vi "CreateRecordingFolder.vi"(0 "Data folder":path, 1 "mouseNumber":i32, 2 "sessionID":string, 4 "Google Drive":bool) -> (5 "Recording Path":path)   [LabVIEW 2013]
panel:
  # "INPUTS"
  # "OUTPUTS"
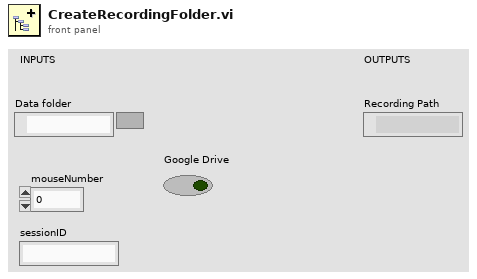
[diagram p1: front panel]
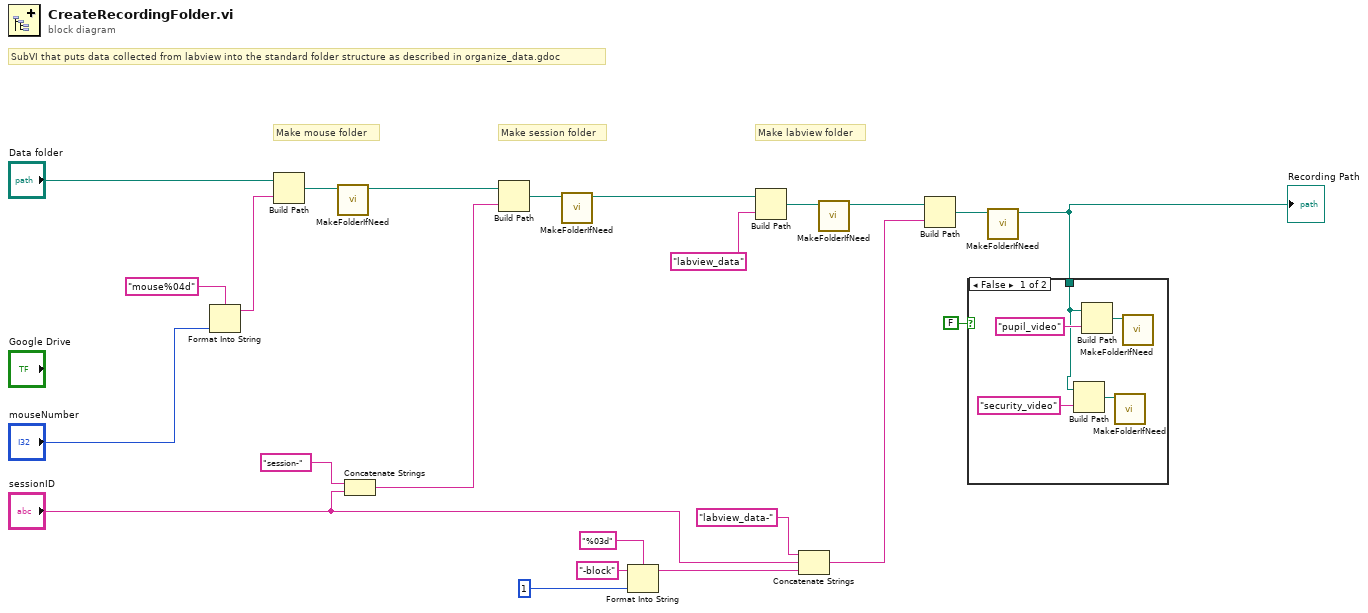
[diagram p0: block diagram]
diagram:
  # "SubVI that puts data collected from labview into the standard folder structure as described in organize_data.gdoc"
  # "Make labview folder"
  # "Make session folder"
  # "Make mouse folder"
  n1 = Format Into String(format string="mouse%04d", "mouseNumber") -> (resulting string=w16:string)  [unwired: 2 in, 1 out]
  n2 = Build Path(base path="Data folder", name or relative path=w16) -> (appended path=w23:path)
  n3 = call "MakeFolderIfNeed.vi"("folder path"=w23) -> ("dup folder path"=w21:path)  [unwired: 10 in]
  n4 = Concatenate Strings("session-" ("string"), "sessionID") -> (w13:string)
  n5 = Build Path(base path=w21, name or relative path=w13) -> (appended path=w22:path)
  n6 = call "MakeFolderIfNeed.vi"("folder path"=w22) -> ("dup folder path"=w19:path)  [unwired: 10 in]
  n7 = Format Into String(format string="%03d", initial string="-block", 1 ("input 1")) -> (resulting string=w10:string)  [unwired: 1 in, 1 out]
  n8 = Build Path(base path=w19, name or relative path="labview_data") -> (appended path=w20:path)
  n9 = Concatenate Strings("labview_data-" ("string"), "sessionID", w10) -> (w4:string)
  n10 = call "MakeFolderIfNeed.vi"("folder path"=w20) -> ("dup folder path"=w3:path)  [unwired: 10 in]
  n11 = Build Path(base path=w3, name or relative path=w4) -> (appended path=w5:path)
  n12 = call "MakeFolderIfNeed.vi"("folder path"=w5) -> ("dup folder path"=w2:path)  [unwired: 10 in]
  "Recording Path" <- w2
  n13 = case shown="False" FALSE {
    tunnel: w2 -> [w24 _]
    frame False {
      n14 = Build Path(base path=w24, name or relative path="security_video") -> (appended path=w26:path)
      n15 = Build Path(base path=w24, name or relative path="pupil_video") -> (appended path=w27:path)
      n16 = call "MakeFolderIfNeed.vi"("folder path"=w26) -> ()  [unwired: 10 in, 1 out]
      n17 = call "MakeFolderIfNeed.vi"("folder path"=w27) -> ()  [unwired: 10 in, 1 out]
    }
    frame True {
    }
  }
